vi "Gyro History Global.vi"(7 "Allocate Size":i32, 8 "error in":errorcluster, 9 "Get ms ago":u32, 10 "Operation":T2, 11 "Gyro":dbl format="%#_13g") -> (0 "error out":errorcluster, 3 "Angle":dbl)   [LabVIEW 2016, in "Path Track.lvlib"]
uses:
  Path Track.lvlib
  FGV Control.ctl
  Gyro History.ctl
panel:
  out "Array":T1[](array[typedef]) {"Timestamp" format="%#_14g"}
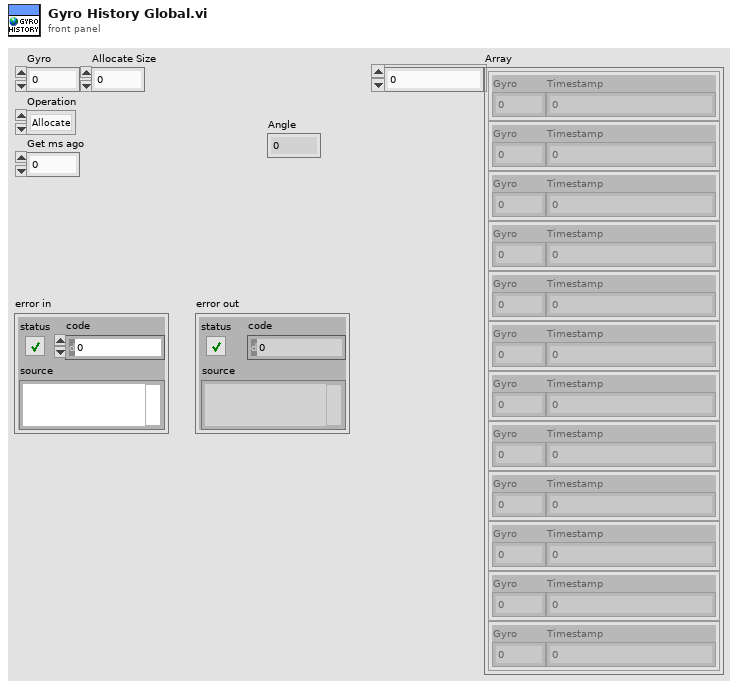
[diagram p1: front panel]
types:
  T1 = typedef "Path Track.lvlib/Gyro History.ctl" = cluster{"Gyro":dbl, "Timestamp":dbl}
  T2 = typedef "Path Track.lvlib/FGV Control.ctl" = enum16{"Allocate", "Get", "Append"}
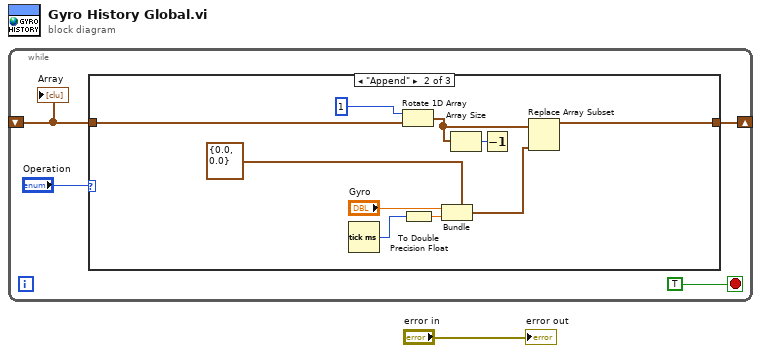
[diagram p0: block diagram]
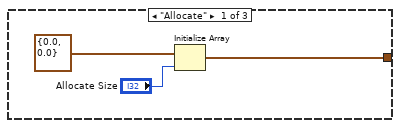
[diagram p2: hidden frame]
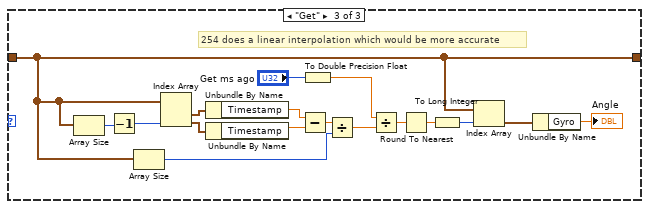
[diagram p3: hidden frame]
diagram:
  n1 = while {
    shift-right: [w3] -> _
    shift-left: _ -> [w2]
    stop <- TRUE stop-if-true
    n2 = case shown="\"Append\"" "Operation" {
      tunnel: [w6 w13 w21] -> w3
      tunnel: w2 -> [_ w15 w21]
      frame "Allocate" {
        n3 = Initialize Array(T1 {"Gyro"=0.0, "Timestamp"=0.0} ("cluster"), "Allocate Size") -> (w6:T1[])
      }
      frame "Append" {
        n4 = Tick Count (ms)() -> (millisecond timer value=w17:u32)
        n5 = Rotate 1D Array(1:w15, 2:1 ("n")) -> (0:w11:T1[])
        n6 = To Double Precision Float(number=w17) -> (double precision float=w12:dbl)
        n7 = Bundle(cluster=T1 {"Gyro"=0.0, "Timestamp"=0.0}, "Gyro"="Gyro", "Timestamp"=w12) -> (w9:T1)
        n8 = Array Size(array=w11) -> (size(s)=w10:i32)
        n9 = Decrement(x=w10) -> ()  [unwired: 1 out]
        n10 = Replace Array Subset(array=w11, new element=w9) -> (w13:T1[])  [unwired: 1 in]
      }
      frame "Get" {
        # "254 does a linear interpolation which would be more accurate"
        n11 = Array Size(array=w21) -> (size(s)=w20:i32)
        n12 = Decrement(x=w20) -> (x-1=w19:i32)
        n13 = Array Size(array=w21) -> (size(s)=w35:i32)
        n14 = Index Array(array=w21, index #2=w19) -> (element #1=w34:T1, element #2=w32:T1)  [unwired: 1 in]
        n15 = Unbundle By Name(w34) -> ("Timestamp"=w31:dbl)
        n16 = Unbundle By Name(w32) -> ("Timestamp"=w30:dbl)
        n17 = Subtract(x=w31, y=w30) -> (x-y=w29:dbl)
        n18 = To Double Precision Float(number="Get ms ago") -> (double precision float=w23:dbl)
        n19 = Divide(x=w29, y=w35) -> (x/y=w24:dbl)
        n20 = Divide(x=w23, y=w24) -> (x/y=w22:dbl)
        n21 = Round To Nearest(number=w22) -> (nearest integer value=w28:dbl)
        n22 = To Long Integer(number=w28) -> (32bit integer=w27:i32)
        n23 = Index Array(array=w21, index=w27) -> (element=w26:T1)
        n24 = Unbundle By Name(w26) -> ("Gyro"=→"Angle":dbl)
      }
    }
    "Array" <- w2
  }
  "error out" <- "error in"
